vi "Drive_Execute.vi"() -> ()   [LabVIEW 2018]
uses:
  Drive_Control_Type.ctl
  <vilib>/Rock Robotics/WPI/ThirdParty/Phoenix-LabVIEW/Motor Controller/Controls/CTRE_Phoenix_MotorControl_ControlMode.ctl
  Global_Variables/Drive_Globals.vi
  Global_Variables/Sensor_Values.vi
  Global_Variables/Climb_Globals.vi
  Global_Variables/Kinematic_Globals.vi
  <vilib>/Utility/file.llb/Write Delimited Spreadsheet (DBL).vi
panel:
  in  "kP_Turn_Target":dbl
  in  "Kd":dbl
  in  "Ki":dbl
  in  "Kp":dbl=0.012
  in  "Turn_Adjust":dbl=0.015
  in  "Max_Linear_Speed":dbl=18.0
  in  "Max_Rotational_Speed":dbl=4.15
  out "Wheel_Speeds":cluster{dbl, dbl, dbl, dbl}(graph)
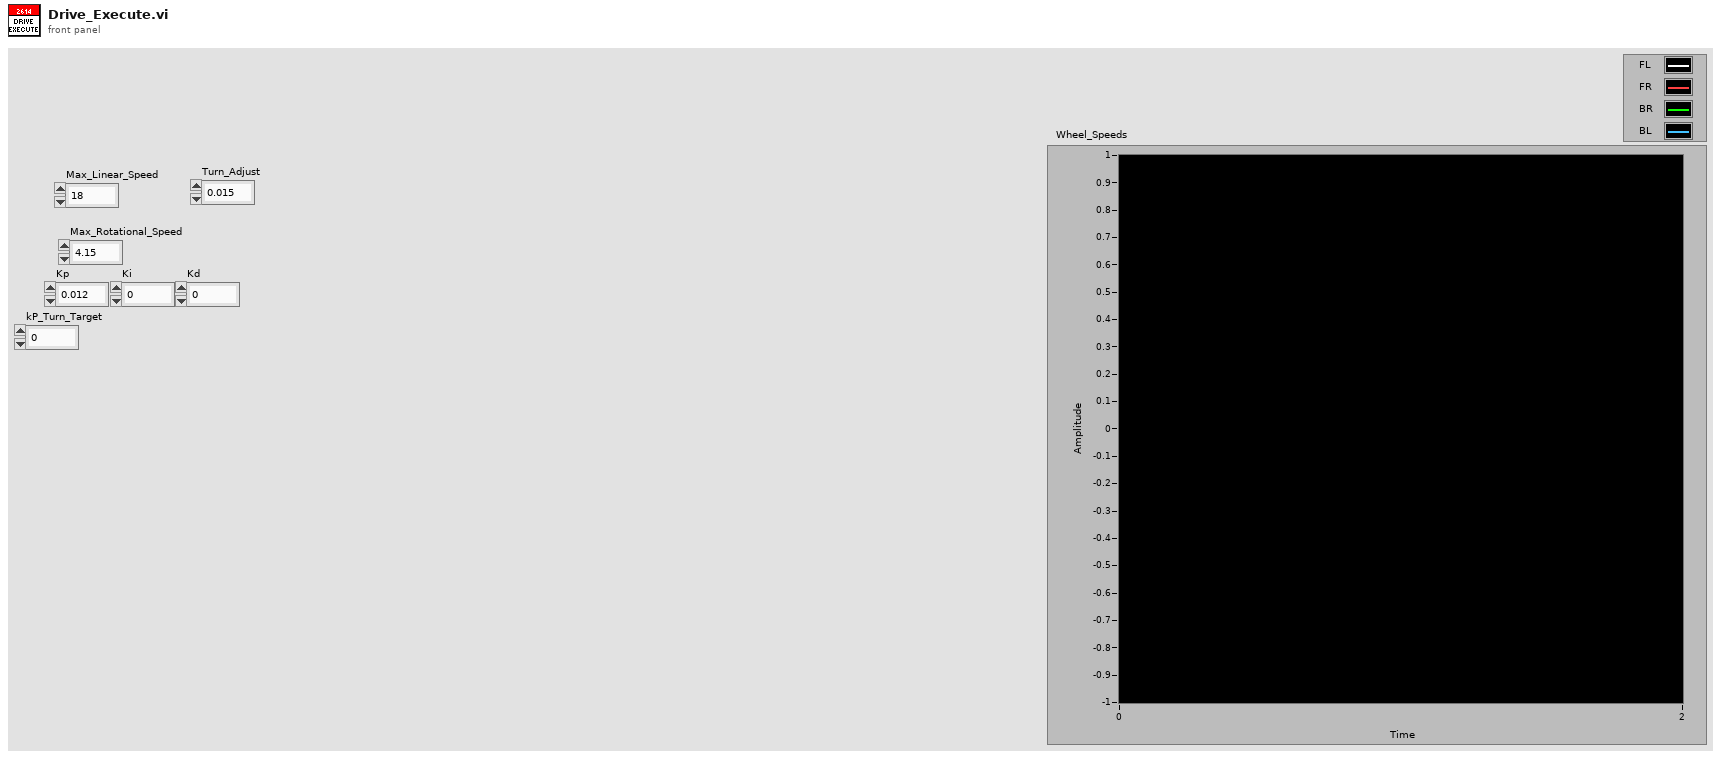
[diagram p1: front panel]
types:
  T1 = typedef "WPI_MotorControlDeviceRef.ctl" = cluster{"DeviceStatus":errorcluster, "Type":T2, "PWM":cluster{"PWM Channel":T3, "DeadBand":T4}, "CAN":cluster{"Device Number":u8, "SetOutput VI Ref":variant, "GetOutput VI Ref":variant, "Enable VI Ref":variant, "Disable VI Ref":variant, "Data":variant}, "Invert":bool, "DIO PWM":cluster{"PWM \"Enable\" Channel":T3, "DIOChannel":T5, "PWM Rate":dbl}}
  T2 = typedef "WPI_MotorControlType.ctl" = enum16{"PWM", "CAN", "DIO PWM"}
  T3 = typedef "FPGA_DIOPWMChannel.ctl" = enum8{"PWM 0", "PWM 1", "PWM 2", "PWM 3", "PWM 4", "PWM 5", "PWM 6", "PWM 7", "PWM 8", "PWM 9", "PWM MXP 0", "PWM MXP 1", "PWM MXP 2", "PWM MXP 3", "PWM MXP 4", "PWM MXP 5", "PWM MXP 6", "PWM MXP 7", "PWM MXP 8", "PWM MXP 9", "Invalid"}
  T4 = typedef "WPI_PWMDeadband.ctl" = cluster{"Name":string, "maxPositivePwm":i32, "minPositivePwm":i32, "centerPwm":i32, "maxNegativePwm":i32, "minNegativePwm":i32, "angularRange":u16}
  T5 = typedef "FPGA_DIOChannel.ctl" = enum8{"DIO 0", "DIO 1", "DIO 2", "DIO 3", "DIO 4", "DIO 5", "DIO 6", "DIO 7", "DIO 8", "DIO 9", "DIO MXP 0", "DIO MXP 1", "DIO MXP 2", "DIO MXP 3", "DIO MXP 4", "DIO MXP 5", "DIO MXP 6", "DIO MXP 7", "DIO MXP 8", "DIO MXP 9", "DIO MXP 10", "DIO MXP 11", "DIO MXP 12", "DIO MXP 13", "DIO MXP 14", "DIO MXP 15", "SPI Port CS1", "SPI Port CS2", "SPI Port CS3", "SPI Port MISO", "SPI Port MOSI", "Invalid"}
  T6 = typedef "CTRE_PigeonIMU_DeviceRef.ctl" = cluster{"DeviceStatus":errorcluster, "Device Number":u8, "Type":T7, "Device ID":u32, "Handle":u64, "UsageFrame":u32, "Library Path":path}
  T7 = typedef "CTRE_PigeonIMU_ConnectionType.ctl" = u32
  T8 = typedef "Drive_Control_Type.ctl" = enum16{"No_Op", "Write_FL_Position", "Write_FR_Position", "Write_BL_Position", "Write_BR_Position", "Set_Encoder_Positions", "Fieldcentric_PercentVBus", "Fieldcentric", "Robotcentric", "Reset_Gyro", "FR_Wheel", "FL_Wheel", "BR_Wheel", "BL_Wheel", "Drive_Onto_Platform", "Manual_Wheel_Control", "Distance", "Turn_To_Heading", "Turn_To_Target", "Drive_To_Target", "Zero", "Auto_Target", "Drive_Over_Platform", "Heading_Lock", "Time"}
  T9 = typedef "Drive_Notifier.ctl" = cluster{"Drive Control List":T8, "Front/Back":dbl, "Left/Right":dbl, "Turn":dbl, "Test_Joy_Y":dbl, "Test_Joy_X":dbl, "Set Wheel Encoder Positions":bool, "Robotcentric":bool, "Reset Gyro":bool, "Rotate Front Right":bool, "Rotate Front Left":bool, "Rotate Back Right":bool, "Rotate Back Left":bool, "Write_Encoder_Positions":bool, "Climb_Advance":bool, "Parameter_One":dbl, "Parameter_Two":dbl, "Parameter_Three":dbl, "Parameter_Four":dbl, "Drive_Notifier":refnum<notifier>, "Step":i32, "Climb_Reverse":bool, "Auto_Target":bool}
  T10 = typedef "CTRE_Phoenix_MotorControl_ControlMode.ctl" = u16
  T11 = cluster{"FL_Out":dbl, "FR_Out":dbl, "BL_Out":dbl, "BR_Out":dbl}
  T12 = cluster{"offsetAngle H":dbl, "offsetAngle V":dbl, "area":dbl, "skew":dbl}
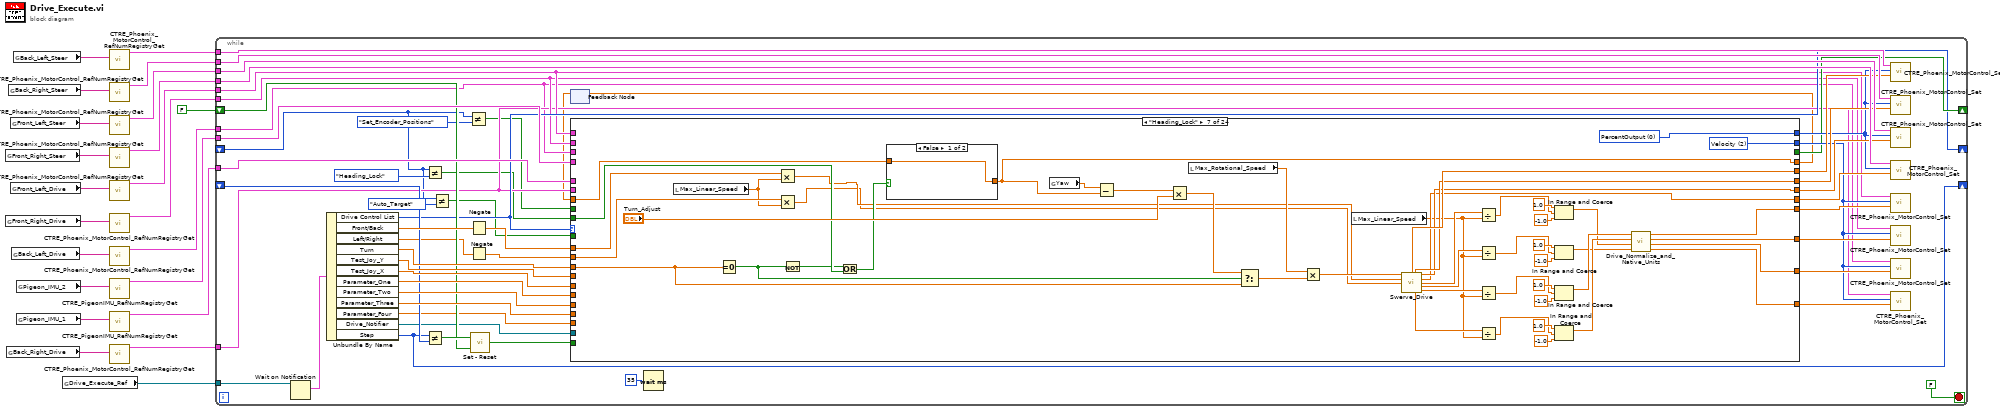
[diagram p0: block diagram]
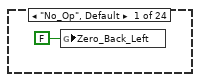
[diagram p2: hidden frame]
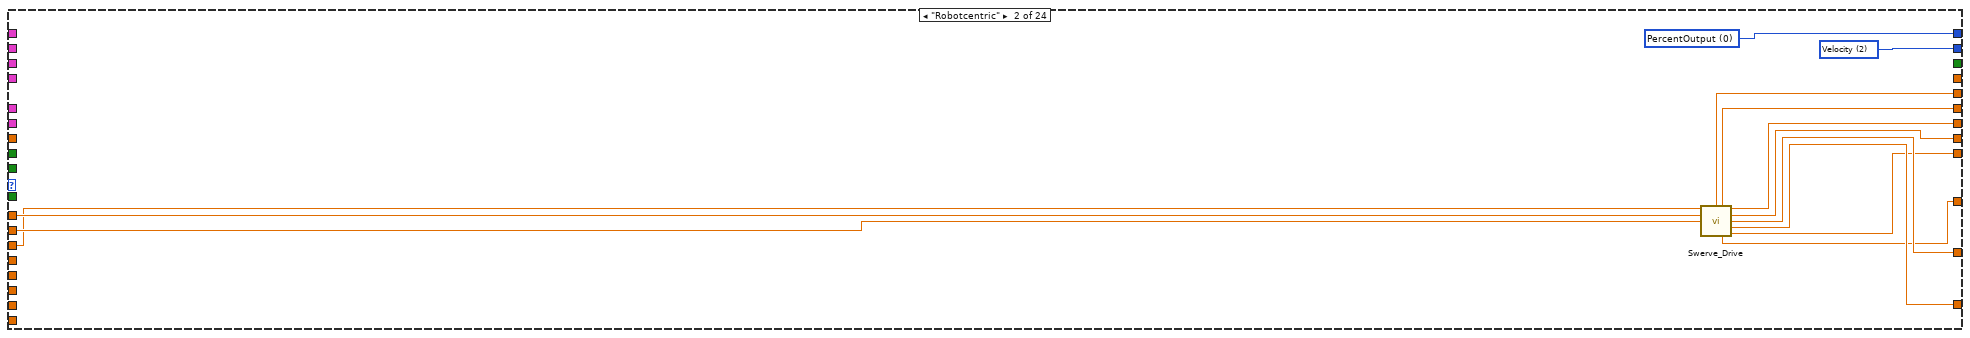
[diagram p3: hidden frame]
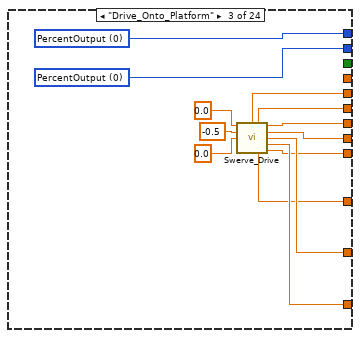
[diagram p4: hidden frame]
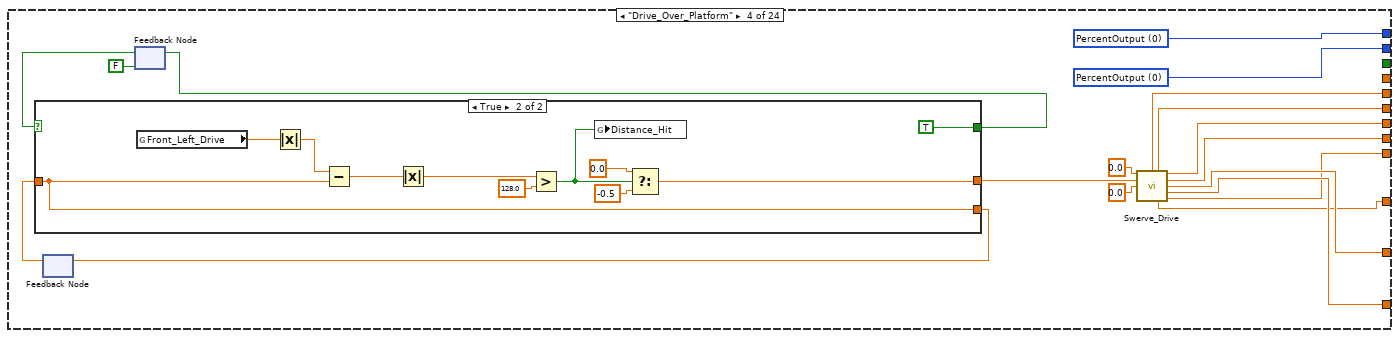
[diagram p5: hidden frame]
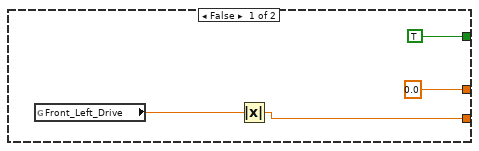
[diagram p6: hidden frame]
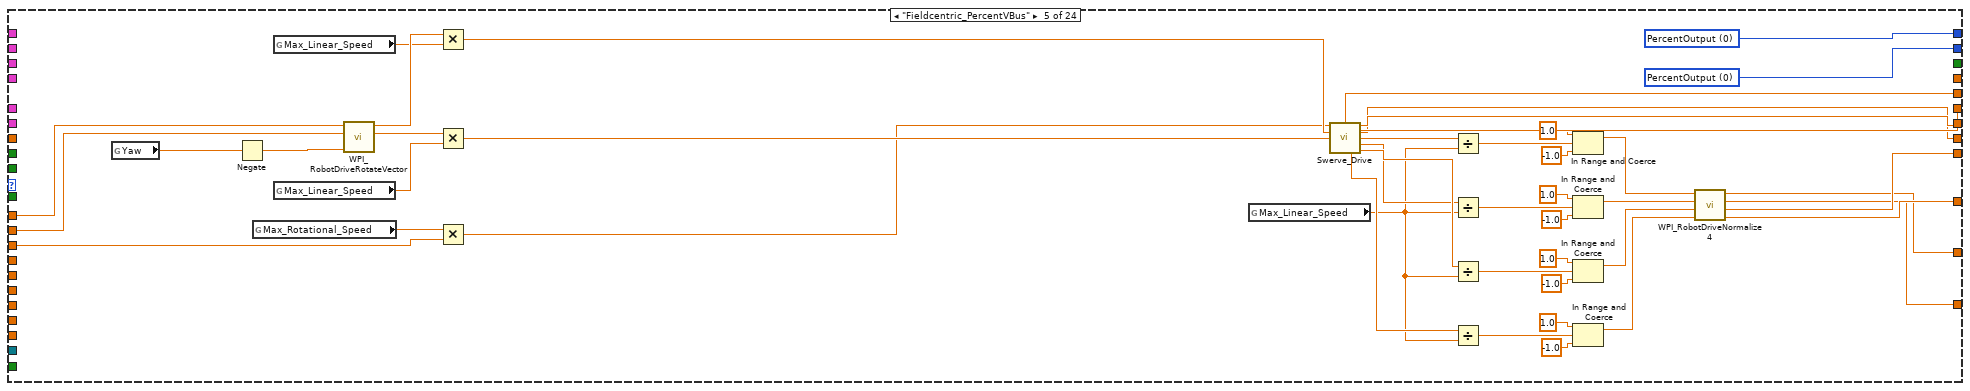
[diagram p7: hidden frame]
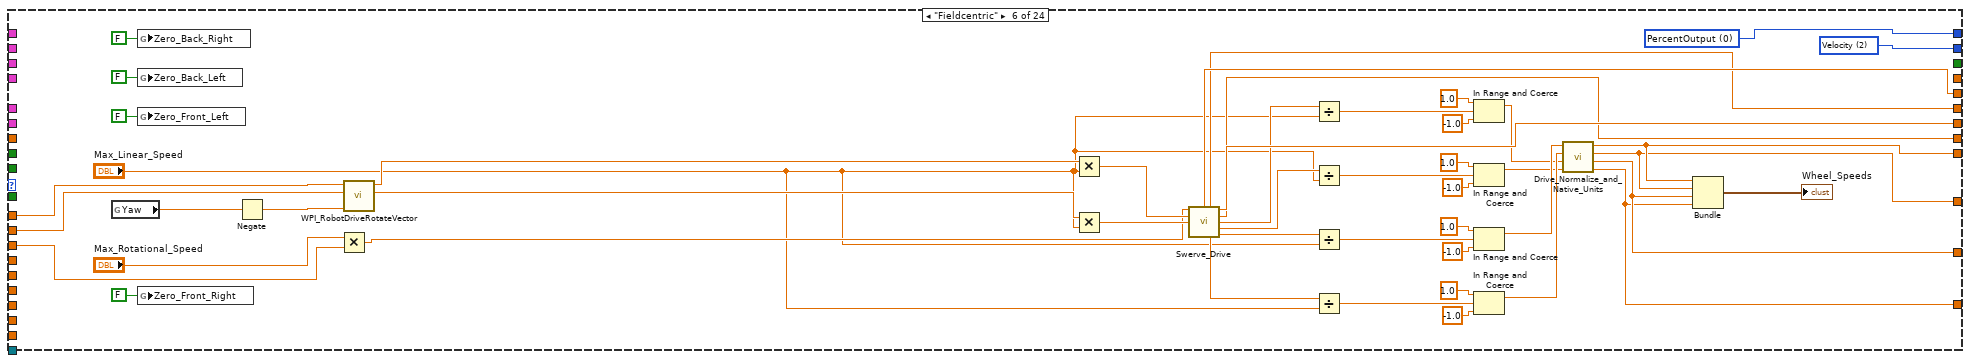
[diagram p8: hidden frame]
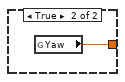
[diagram p9: hidden frame]
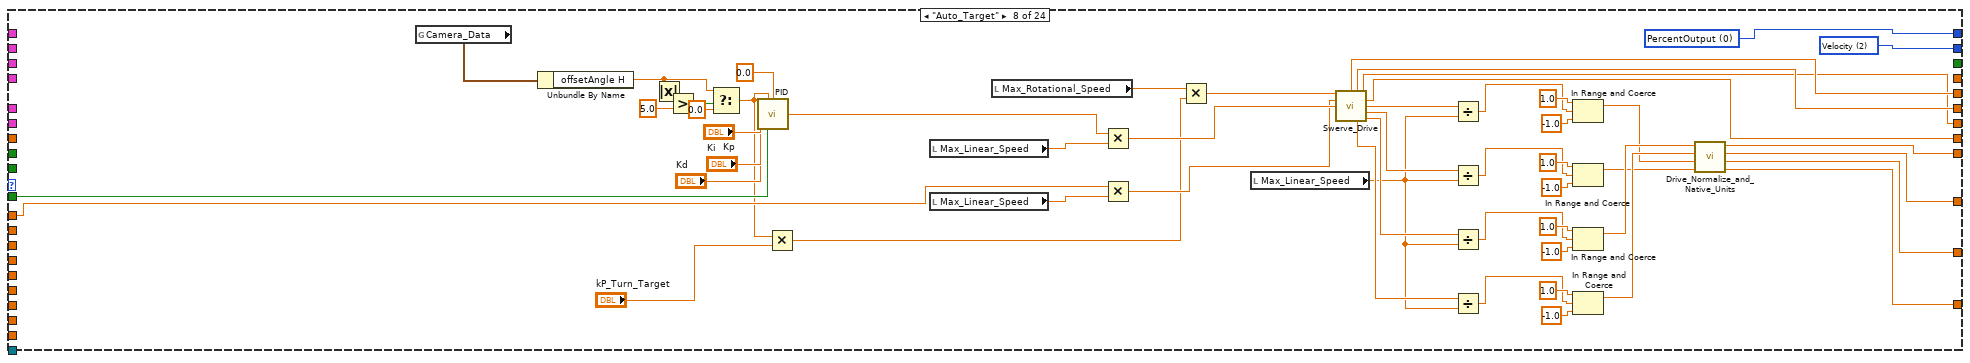
[diagram p10: hidden frame]
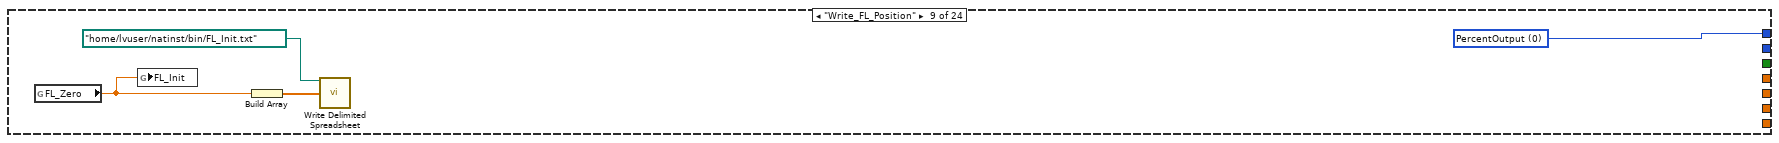
[diagram p11: hidden frame]
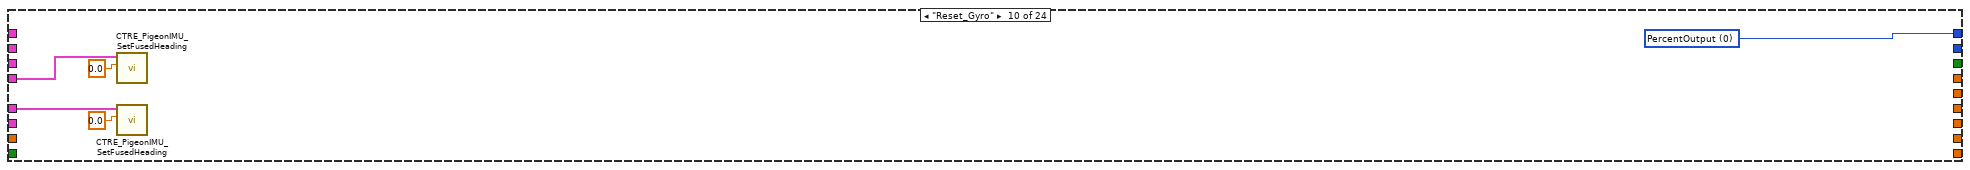
[diagram p12: hidden frame]
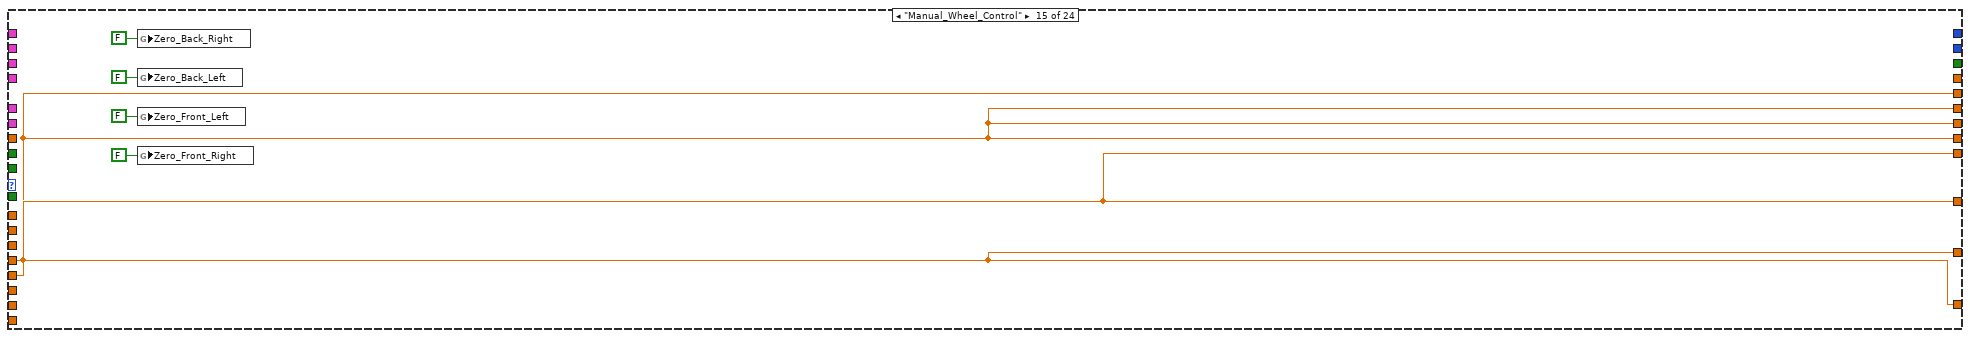
[diagram p17: hidden frame]
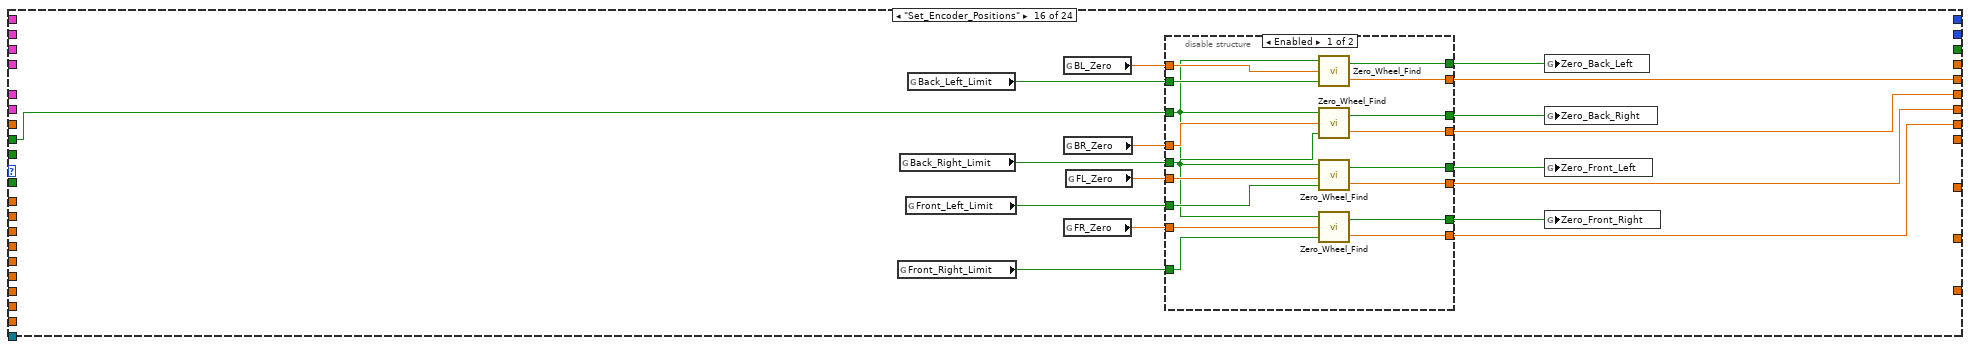
[diagram p18: hidden frame]
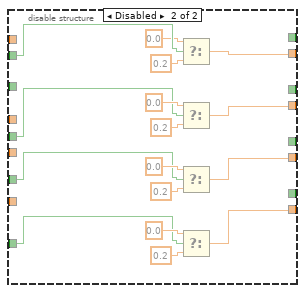
[diagram p19: hidden frame]
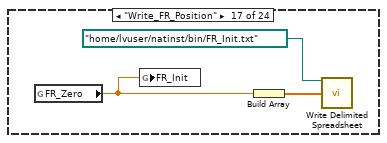
[diagram p20: hidden frame]
diagram:
  n1 = global read "Drive_Globals.vi" "Front_Right_Steer"() -> (w7:string)
  n2 = global read "Drive_Globals.vi" "Front_Right_Drive"() -> (w12:string)
  n3 = global read "Drive_Globals.vi" "Back_Right_Drive"() -> (w10:string)
  n4 = global read "Drive_Globals.vi" "Back_Right_Steer"() -> (w5:string)
  n5 = global read "Drive_Globals.vi" "Front_Left_Steer"() -> (w6:string)
  n6 = global read "Drive_Globals.vi" "Front_Left_Drive"() -> (w11:string)
  n7 = global read "Drive_Globals.vi" "Back_Left_Drive"() -> (w9:string)
  n8 = global read "Drive_Globals.vi" "Back_Left_Steer"() -> (w8:string)
  n9 = global read "Drive_Globals.vi" "Pigeon_IMU_2"() -> (w3:string)
  n10 = global read "Drive_Globals.vi" "Pigeon_IMU_1"() -> (w4:string)
  n11 = global read "Drive_Globals.vi" "Drive_Execute_Ref"() -> (w22:refnum<notifier>)
  n12 = call <vilib>:"CTRE_Phoenix_MotorControl_RefNumRegistryGet.vi"("refnum name"=w8) -> ("PhoenixMotorControlDevRef"=w17:T1)  [unwired: 9 in, 1 out]
  n13 = call <vilib>:"CTRE_Phoenix_MotorControl_RefNumRegistryGet.vi"("refnum name"=w5) -> ("PhoenixMotorControlDevRef"=w14:T1)  [unwired: 9 in, 1 out]
  n14 = call <vilib>:"CTRE_Phoenix_MotorControl_RefNumRegistryGet.vi"("refnum name"=w6) -> ("PhoenixMotorControlDevRef"=w15:T1)  [unwired: 9 in, 1 out]
  n15 = call <vilib>:"CTRE_Phoenix_MotorControl_RefNumRegistryGet.vi"("refnum name"=w7) -> ("PhoenixMotorControlDevRef"=w16:T1)  [unwired: 9 in, 1 out]
  n16 = call <vilib>:"CTRE_Phoenix_MotorControl_RefNumRegistryGet.vi"("refnum name"=w11) -> ("PhoenixMotorControlDevRef"=w20:T1)  [unwired: 9 in, 1 out]
  n17 = call <vilib>:"CTRE_Phoenix_MotorControl_RefNumRegistryGet.vi"("refnum name"=w12) -> ("PhoenixMotorControlDevRef"=w21:T1)  [unwired: 9 in, 1 out]
  n18 = call <vilib>:"CTRE_Phoenix_MotorControl_RefNumRegistryGet.vi"("refnum name"=w9) -> ("PhoenixMotorControlDevRef"=w19:T1)  [unwired: 9 in, 1 out]
  n19 = call <vilib>:"CTRE_PigeonIMU_RefNumRegistryGet.vi"("refnum name"=w3) -> ("PigeonIMUDevRef"=w2:T6)  [unwired: 9 in, 1 out]
  n20 = call <vilib>:"CTRE_PigeonIMU_RefNumRegistryGet.vi"("refnum name"=w4) -> ("PigeonIMUDevRef"=w13:T6)  [unwired: 9 in, 1 out]
  n21 = call <vilib>:"CTRE_Phoenix_MotorControl_RefNumRegistryGet.vi"("refnum name"=w10) -> ("PhoenixMotorControlDevRef"=w18:T1)  [unwired: 9 in, 1 out]
  n22 = while {
    tunnel: w22 -> [w54]
    tunnel: w21 -> [w36]
    tunnel: w20 -> [w37]
    tunnel: w19 -> [w34]
    tunnel: w18 -> [w35]
    tunnel: w14 -> [w71]
    tunnel: w17 -> [w58]
    tunnel: w16 -> [w70]
    tunnel: w15 -> [w69]
    tunnel: w13 -> [w57]
    tunnel: w2 -> [w51]
    shift-right: [w38] -> _
    shift-left: _ -> [w25]
    shift-right: [w43] -> _
    shift-left: _ -> [w44]
    shift-right: [w47] -> _
    shift-left: FALSE ("Reinit") -> [w45]
    stop <- FALSE stop-if-true
    n23 = Wait on Notification(notifier=w54) -> (notification=w40:T9)  [unwired: 3 in, 3 out]
    n24 = Unbundle By Name(w40) -> ("Drive Control List"=w38:T8, "Front/Back"=w72:dbl, "Left/Right"=w33:dbl, "Turn"=w68:dbl, "Test_Joy_Y"=w56:dbl, "Test_Joy_X"=w53:dbl, "Parameter_One"=w50:dbl, "Parameter_Two"=w48:dbl, "Parameter_Three"=w49:dbl, "Parameter_Four"=w39:dbl, "Drive_Notifier"=w41:refnum<notifier>, "Step"=w43:i32)
    n25 = Not Equal?(x=w25, y=Drive_Control_Type."Heading_Lock") -> (x != y?=w26:bool)
    n26 = Not Equal?(x=w43, y=w44) -> (x != y?=w46:bool)
    n27 = Not Equal?(x=w25, y=Drive_Control_Type."Auto_Target") -> (x != y?=w23:bool)
    n28 = Not Equal?(x=w25, y=Drive_Control_Type."Set_Encoder_Positions") -> (x != y?=w30:bool)
    n29 = Negate(x=w72) -> (-x=w52:dbl)
    n30 = Negate(x=w33) -> (-x=w32:dbl)
    n31 = call "Set - Reset.vi"("Reset"=w45, "Set"=w46) -> ("Output"=w42:bool)
    n32 = feedback #1() -> (w29:dbl)  [unwired: 1 in]
    n33 = case shown="\"Heading_Lock\"" w38 {
      tunnel: w52 -> [_ w78 _ _ w171 w218 w243 w285 _ _ _ _ _ _ _ _ _ _ _ _ _ _ _ _]
      tunnel: w32 -> [_ w79 _ _ w170 w217 w242 _ _ _ _ _ _ _ _ _ _ _ _ _ _ _ _ _]
      tunnel: w68 -> [_ w76 _ _ w143 w194 w234 _ _ _ _ _ _ _ _ _ _ _ _ _ _ _ _ _]
      tunnel: [_ w87 w100 w118 w177 w224 w274 w329 _ _ _ _ _ w346 w352 w370 _ _ _ w427 w452 w464 w478 w495] -> w67
      tunnel: [_ w83 w96 w114 w135 w186 w246 w301 _ _ _ _ _ w347 w353 _ _ _ _ w418 w445 w460 w474 w491] -> w66
      tunnel: [_ w86 w99 w117 w176 w223 w273 w328 _ _ _ _ w345 _ w352 w363 _ _ _ w426 w451 w463 w477 w494] -> w65
      tunnel: [_ w82 w95 w113 w136 w185 w245 w300 _ _ _ _ w344 _ w353 _ _ _ _ w420 w447 w459 w473 w490] -> w64
      tunnel: [_ w84 w97 w115 w174 w221 w271 w326 _ _ w341 _ _ _ w352 w354 _ _ _ w424 w449 w461 w475 w492] -> w63
      tunnel: [_ w80 w93 w111 w138 w187 w247 w302 _ _ w340 _ _ _ w353 _ _ _ _ w414 w441 w457 w471 w488] -> w62
      tunnel: [_ w85 w98 w116 w175 w222 w272 w327 _ _ _ w342 _ _ w352 w359 _ _ _ w425 w450 w462 w476 w493] -> w61
      tunnel: [_ w81 w94 w112 w137 w188 w248 w303 _ _ _ w343 _ _ w353 _ _ _ _ w416 w443 w458 w472 w489] -> w60
      tunnel: [_ w88 w101 w119 w178 w225 w275 w330 w334 w339 _ _ _ _ _ _ _ _ _ _ _ _ _ _] -> w59
      tunnel: w57 -> [_ _ _ _ _ _ _ _ _ w338 _ _ _ _ _ _ _ _ _ _ _ _ _ _]
      tunnel: w56 -> [_ _ _ _ _ _ _ _ _ _ w340 w343 w344 w347 w353 _ _ _ _ _ _ _ _ _]
      tunnel: [_ w77 w92 w110 w173 w220 w270 w325 _ _ _ _ _ _ _ _ _ _ _ w413 w440 w454 _ w486] -> w55
      tunnel: w53 -> [_ _ _ _ _ _ _ _ _ _ w341 w342 w345 w346 w352 _ _ _ _ _ _ _ _ _]
      tunnel: w51 -> [_ _ _ _ _ _ _ _ _ w335 _ _ _ _ _ _ _ _ _ _ _ _ _ _]
      tunnel: w50 -> [_ _ _ _ _ _ _ _ _ _ _ _ _ _ _ _ _ _ _ _ w433 w455 _ w485]
      tunnel: w49 -> [_ _ _ _ _ _ _ _ _ _ _ _ _ _ _ _ _ _ _ w422 _ _ _ _]
      tunnel: w48 -> [_ _ _ _ _ _ _ _ _ _ _ _ _ _ _ _ _ _ _ _ w434 _ _ w484]
      tunnel: [_ _ _ _ _ _ _ _ _ _ _ _ _ _ _ _ _ _ _ w432 w437 w469 w483 w500] -> w47
      tunnel: w42 -> [_ _ _ _ _ _ _ _ _ _ _ _ _ _ _ _ _ _ _ w431 w436 w468 w482 w499]
      tunnel: w41 -> [_ _ _ _ _ _ _ _ _ _ _ _ _ _ _ _ _ _ _ w429 w453 w466 w480 w497]
      tunnel: w39 -> [_ _ _ _ _ _ _ _ _ _ _ _ _ _ _ _ _ _ _ w423 w435 w456 w470 w487]
      tunnel: w37 -> [_ _ _ _ _ _ _ _ _ _ _ _ _ _ _ _ _ _ _ _ _ _ _ _]
      tunnel: w36 -> [_ _ _ _ _ _ _ _ _ _ _ _ _ _ _ _ _ _ _ _ _ _ _ _]
      tunnel: w35 -> [_ _ _ _ _ _ _ _ _ _ _ _ _ _ _ _ _ _ _ _ _ _ _ _]
      tunnel: w34 -> [_ _ _ _ _ _ _ _ _ _ _ _ _ _ _ _ _ _ _ _ _ _ _ _]
      tunnel: w30 -> [_ _ _ _ _ _ _ _ _ _ _ _ _ _ _ w355 _ _ _ _ _ _ _ _]
      tunnel: w29 -> [_ _ _ _ _ _ w236 _ _ _ _ _ _ _ _ _ _ _ _ _ _ _ _ _]
      tunnel: w26 -> [_ _ _ _ _ _ w237 _ _ _ _ _ _ _ _ _ _ _ _ _ _ _ _ _]
      tunnel: [_ _ _ _ _ _ w235 _ _ _ _ _ _ _ _ _ _ _ _ _ _ _ _ _] -> w27
      tunnel: w23 -> [_ _ _ _ _ _ _ w297 _ _ _ _ _ _ _ _ _ _ _ _ _ _ _ _]
      frame "No_Op", Default {
        n34 = global write "Drive_Globals.vi" "Zero_Back_Left"(FALSE ("Zero_Back_Left")) -> ()
      }
      frame "Robotcentric" {
        w77 = T10 2 items=["PercentOutput"=0, "Position"=1, "Velocity"=2, "Current"=3, "Follower"=5, "MotionProfile"=6, "MotionMagic"=7, "MotionMagicArc"=8, "MotionProfileArc"=10, "Disabled"=15] ("Control Mode")
        w88 = T10 0 items=["PercentOutput"=0, "Position"=1, "Velocity"=2, "Current"=3, "Follower"=5, "MotionProfile"=6, "MotionMagic"=7, "MotionMagicArc"=8, "MotionProfileArc"=10, "Disabled"=15] ("Control Mode")
        n35 = call "Swerve_Drive.vi"("Z"=w76, "Y"=w78, "X"=w79) -> ("Back Left Spin Speed"=w87:dbl, "Back Right Spin Speed"=w86:dbl, "Front Left Spin Speed"=w85:dbl, "Front Right Spin Speed"=w84:dbl, "Back Left Motor Power"=w83:dbl, "Back Right Motor Power"=w82:dbl, "Front Right Motor Power"=w80:dbl, "Front Left Motor Power"=w81:dbl)  [unwired: 5 in]
      }
      frame "Drive_Onto_Platform" {
        w92 = T10 0 items=["PercentOutput"=0, "Position"=1, "Velocity"=2, "Current"=3, "Follower"=5, "MotionProfile"=6, "MotionMagic"=7, "MotionMagicArc"=8, "MotionProfileArc"=10, "Disabled"=15] ("Control Mode")
        w101 = T10 0 items=["PercentOutput"=0, "Position"=1, "Velocity"=2, "Current"=3, "Follower"=5, "MotionProfile"=6, "MotionMagic"=7, "MotionMagicArc"=8, "MotionProfileArc"=10, "Disabled"=15] ("Control Mode")
        n36 = call "Swerve_Drive.vi"("Z"=0.0, "Y"=-0.5, "X"=0.0) -> ("Back Left Spin Speed"=w100:dbl, "Back Right Spin Speed"=w99:dbl, "Front Left Spin Speed"=w98:dbl, "Front Right Spin Speed"=w97:dbl, "Back Left Motor Power"=w96:dbl, "Back Right Motor Power"=w95:dbl, "Front Right Motor Power"=w93:dbl, "Front Left Motor Power"=w94:dbl)  [unwired: 5 in]
      }
      frame "Drive_Over_Platform" {
        w110 = T10 0 items=["PercentOutput"=0, "Position"=1, "Velocity"=2, "Current"=3, "Follower"=5, "MotionProfile"=6, "MotionMagic"=7, "MotionMagicArc"=8, "MotionProfileArc"=10, "Disabled"=15] ("Control Mode")
        w119 = T10 0 items=["PercentOutput"=0, "Position"=1, "Velocity"=2, "Current"=3, "Follower"=5, "MotionProfile"=6, "MotionMagic"=7, "MotionMagicArc"=8, "MotionProfileArc"=10, "Disabled"=15] ("Control Mode")
        n37 = feedback #2() -> (w102:dbl)  [unwired: 1 in]
        n38 = feedback #3(FALSE) -> (w107:bool)
        n39 = case shown="True" w107 {
          tunnel: [TRUE TRUE] -> w105
          tunnel: [0.0 ("Y") w126] -> w104
          tunnel: [w120 w128] -> w103
          tunnel: w102 -> [_ w128]
          frame False {
            n40 = global read "Sensor_Values.vi" "Front_Left_Drive"() -> (w121:dbl)
            n41 = Absolute Value(x=w121) -> (abs(x)=w120:dbl)
          }
          frame True {
            n42 = global read "Sensor_Values.vi" "Front_Left_Drive"() -> (w133:dbl)
            n43 = Absolute Value(x=w133) -> (abs(x)=w132:dbl)
            n44 = Subtract(x=w132, y=w128) -> (x-y=w131:dbl)
            n45 = Absolute Value(x=w131) -> (abs(x)=w130:dbl)
            n46 = Greater?(x=w130, y=128.0) -> (0:w124:bool)
            n47 = global write "Climb_Globals.vi" "Distance_Hit"(w124) -> ()
            n48 = Select(t=0.0, s=w124, f=-0.5 ("Y")) -> (s? t:f=w126:dbl)
          }
        }
        n49 = feedback-in #2(w103) -> ()
        n50 = feedback-in #3(w105) -> ()
        n51 = call "Swerve_Drive.vi"("Z"=0.0, "Y"=w104, "X"=0.0) -> ("Back Left Spin Speed"=w118:dbl, "Back Right Spin Speed"=w117:dbl, "Front Left Spin Speed"=w116:dbl, "Front Right Spin Speed"=w115:dbl, "Back Left Motor Power"=w114:dbl, "Back Right Motor Power"=w113:dbl, "Front Right Motor Power"=w111:dbl, "Front Left Motor Power"=w112:dbl)  [unwired: 5 in]
      }
      frame "Fieldcentric_PercentVBus" {
        w173 = T10 0 items=["PercentOutput"=0, "Position"=1, "Velocity"=2, "Current"=3, "Follower"=5, "MotionProfile"=6, "MotionMagic"=7, "MotionMagicArc"=8, "MotionProfileArc"=10, "Disabled"=15] ("Control Mode")
        w178 = T10 0 items=["PercentOutput"=0, "Position"=1, "Velocity"=2, "Current"=3, "Follower"=5, "MotionProfile"=6, "MotionMagic"=7, "MotionMagicArc"=8, "MotionProfileArc"=10, "Disabled"=15] ("Control Mode")
        n52 = global read "Sensor_Values.vi" "Yaw"() -> (w172:dbl)
        n53 = Negate(x=w172) -> (-x=w169:dbl)
        n54 = global read "Kinematic_Globals.vi" "Max_Rotational_Speed"() -> (w145:dbl)
        n55 = global read "Kinematic_Globals.vi" "Max_Linear_Speed"() -> (w146:dbl)
        n56 = global read "Kinematic_Globals.vi" "Max_Linear_Speed"() -> (w151:dbl)
        n57 = call <vilib>:"WPI_RobotDriveRotateVector.vi"("Angle"=w169, "X"=w170, "Y"=w171) -> ("X'"=w150:dbl, "Y'"=w147:dbl)  [unwired: 7 out]
        n58 = Multiply(x=w147, y=w146) -> (x*y=w148:dbl)
        n59 = Multiply(x=w150, y=w151) -> (x*y=w149:dbl)
        n60 = Multiply(x=w145, y=w143) -> (x*y=w144:dbl)
        n61 = global read "Kinematic_Globals.vi" "Max_Linear_Speed"() -> (w152:dbl)
        n62 = call "Swerve_Drive.vi"("Z"=w144, "Y"=w148, "X"=w149) -> ("Back Left Spin Speed"=w177:dbl, "Back Right Spin Speed"=w176:dbl, "Front Left Spin Speed"=w175:dbl, "Front Right Spin Speed"=w174:dbl, "Back Left Motor Power"=w153:dbl, "Back Right Motor Power"=w158:dbl, "Front Right Motor Power"=w161:dbl, "Front Left Motor Power"=w166:dbl)  [unwired: 5 in]
        n63 = Divide(x=w153, y=w152) -> (x/y=w155:dbl)
        n64 = Divide(x=w158, y=w152) -> (x/y=w154:dbl)
        n65 = Divide(x=w166, y=w152) -> (x/y=w165:dbl)
        n66 = Divide(x=w161, y=w152) -> (x/y=w162:dbl)
        n67 = In Range and Coerce(upper limit=1.0, x=w155, lower limit=-1.0) -> (coerced(x)=w139:dbl)  [unwired: 1 out]
        n68 = In Range and Coerce(upper limit=1.0, x=w154, lower limit=-1.0) -> (coerced(x)=w140:dbl)  [unwired: 1 out]
        n69 = In Range and Coerce(upper limit=1.0, x=w165, lower limit=-1.0) -> (coerced(x)=w141:dbl)  [unwired: 1 out]
        n70 = In Range and Coerce(upper limit=1.0, x=w162, lower limit=-1.0) -> (coerced(x)=w142:dbl)  [unwired: 1 out]
        n71 = call <vilib>:"WPI_RobotDriveNormalize 4.vi"("D"=w142, "C"=w141, "B"=w140, "A"=w139) -> ("D'"=w138:dbl, "C'"=w137:dbl, "B'"=w136:dbl, "A'"=w135:dbl)
      }
      frame "Fieldcentric" {
        w220 = T10 2 items=["PercentOutput"=0, "Position"=1, "Velocity"=2, "Current"=3, "Follower"=5, "MotionProfile"=6, "MotionMagic"=7, "MotionMagicArc"=8, "MotionProfileArc"=10, "Disabled"=15] ("Control Mode")
        w225 = T10 0 items=["PercentOutput"=0, "Position"=1, "Velocity"=2, "Current"=3, "Follower"=5, "MotionProfile"=6, "MotionMagic"=7, "MotionMagicArc"=8, "MotionProfileArc"=10, "Disabled"=15] ("Control Mode")
        n72 = global read "Sensor_Values.vi" "Yaw"() -> (w219:dbl)
        n73 = global write "Drive_Globals.vi" "Zero_Back_Right"(FALSE ("Zero_Back_Left")) -> ()
        n74 = global write "Drive_Globals.vi" "Zero_Back_Left"(FALSE ("Zero_Back_Left")) -> ()
        n75 = global write "Drive_Globals.vi" "Zero_Front_Left"(FALSE ("Zero_Back_Left")) -> ()
        n76 = global write "Drive_Globals.vi" "Zero_Front_Right"(FALSE ("Zero_Back_Left")) -> ()
        n77 = Negate(x=w219) -> (-x=w216:dbl)
        n78 = Multiply(x="Max_Rotational_Speed", y=w194) -> (x*y=w195:dbl)
        n79 = call <vilib>:"WPI_RobotDriveRotateVector.vi"("Angle"=w216, "X"=w217, "Y"=w218) -> ("X'"=w199:dbl, "Y'"=w196:dbl)  [unwired: 7 out]
        n80 = Multiply(x=w196, y="Max_Linear_Speed") -> (x*y=w197:dbl)
        n81 = Multiply(x=w199, y="Max_Linear_Speed") -> (x*y=w198:dbl)
        n82 = call "Swerve_Drive.vi"("Z"=w195, "Y"=w197, "X"=w198) -> ("Back Left Spin Speed"=w224:dbl, "Back Right Spin Speed"=w223:dbl, "Front Left Spin Speed"=w222:dbl, "Front Right Spin Speed"=w221:dbl, "Back Left Motor Power"=w200:dbl, "Back Right Motor Power"=w205:dbl, "Front Right Motor Power"=w208:dbl, "Front Left Motor Power"=w213:dbl)  [unwired: 5 in]
        n83 = Divide(x=w200, y="Max_Linear_Speed") -> (x/y=w202:dbl)
        n84 = Divide(x=w205, y="Max_Linear_Speed") -> (x/y=w201:dbl)
        n85 = Divide(x=w213, y="Max_Linear_Speed") -> (x/y=w212:dbl)
        n86 = Divide(x=w208, y="Max_Linear_Speed") -> (x/y=w209:dbl)
        n87 = In Range and Coerce(upper limit=1.0, x=w202, lower limit=-1.0) -> (coerced(x)=w190:dbl)  [unwired: 1 out]
        n88 = In Range and Coerce(upper limit=1.0, x=w201, lower limit=-1.0) -> (coerced(x)=w191:dbl)  [unwired: 1 out]
        n89 = In Range and Coerce(upper limit=1.0, x=w212, lower limit=-1.0) -> (coerced(x)=w193:dbl)  [unwired: 1 out]
        n90 = In Range and Coerce(upper limit=1.0, x=w209, lower limit=-1.0) -> (coerced(x)=w192:dbl)  [unwired: 1 out]
        n91 = call "Drive_Normalize_and_Native_Units.vi"("BR"=w191, "BL"=w190, "FR"=w192, "FL"=w193) -> ("BR_Out"=w185:dbl, "BL_Out"=w186:dbl, "FR_Out"=w187:dbl, "FL_Out"=w188:dbl)
        n92 = Bundle("FL_Out"=w188, "FR_Out"=w187, "BL_Out"=w186, "BR_Out"=w185) -> (→"Wheel_Speeds":T11)  [unwired: 1 in]
      }
      frame "Heading_Lock" {
        w270 = T10 2 items=["PercentOutput"=0, "Position"=1, "Velocity"=2, "Current"=3, "Follower"=5, "MotionProfile"=6, "MotionMagic"=7, "MotionMagicArc"=8, "MotionProfileArc"=10, "Disabled"=15] ("Control Mode")
        w275 = T10 0 items=["PercentOutput"=0, "Position"=1, "Velocity"=2, "Current"=3, "Follower"=5, "MotionProfile"=6, "MotionMagic"=7, "MotionMagicArc"=8, "MotionProfileArc"=10, "Disabled"=15] ("Control Mode")
        n93 = local read "Max_Linear_Speed"() -> (w228:dbl)
        n94 = Equal To 0?(x=w234) -> (x = 0?=w231:bool)
        n95 = Multiply(x=w243, y=w228) -> (x*y=w227:dbl)
        n96 = Multiply(x=w242, y=w228) -> (x*y=w226:dbl)
        n97 = Not(x=w231) -> (.not. x?=w230:bool)
        n98 = Or(x=w230, y=w237) -> (x .or. y?=w232:bool)
        n99 = case shown="False" w232 {
          tunnel: [w276 w277] -> w235
          tunnel: w236 -> [w276 _]
          frame False {
          }
          frame True {
            n100 = global read "Sensor_Values.vi" "Yaw"() -> (w277:dbl)
          }
        }
        n101 = global read "Sensor_Values.vi" "Yaw"() -> (w240:dbl)
        n102 = Subtract(x=w240, y=w235) -> (x-y=w239:dbl)
        n103 = Multiply(x=w239, y="Turn_Adjust") -> (x*y=w241:dbl)
        n104 = local read "Max_Rotational_Speed"() -> (w244:dbl)
        n105 = Select(t=w241, s=w231, f=w234) -> (s? t:f=w233:dbl)
        n106 = Multiply(x=w244, y=w233) -> (x*y=w253:dbl)
        n107 = local read "Max_Linear_Speed"() -> (w229:dbl)
        n108 = call "Swerve_Drive.vi"("Z"=w253, "Y"=w227, "X"=w226) -> ("Back Left Spin Speed"=w274:dbl, "Back Right Spin Speed"=w273:dbl, "Front Left Spin Speed"=w272:dbl, "Front Right Spin Speed"=w271:dbl, "Back Left Motor Power"=w254:dbl, "Back Right Motor Power"=w259:dbl, "Front Right Motor Power"=w262:dbl, "Front Left Motor Power"=w267:dbl)  [unwired: 5 in]
        n109 = Divide(x=w254, y=w229) -> (x/y=w256:dbl)
        n110 = Divide(x=w259, y=w229) -> (x/y=w255:dbl)
        n111 = Divide(x=w267, y=w229) -> (x/y=w266:dbl)
        n112 = Divide(x=w262, y=w229) -> (x/y=w263:dbl)
        n113 = In Range and Coerce(upper limit=1.0, x=w256, lower limit=-1.0) -> (coerced(x)=w249:dbl)  [unwired: 1 out]
        n114 = In Range and Coerce(upper limit=1.0, x=w255, lower limit=-1.0) -> (coerced(x)=w250:dbl)  [unwired: 1 out]
        n115 = In Range and Coerce(upper limit=1.0, x=w266, lower limit=-1.0) -> (coerced(x)=w252:dbl)  [unwired: 1 out]
        n116 = In Range and Coerce(upper limit=1.0, x=w263, lower limit=-1.0) -> (coerced(x)=w251:dbl)  [unwired: 1 out]
        n117 = call "Drive_Normalize_and_Native_Units.vi"("BR"=w250, "BL"=w249, "FR"=w251, "FL"=w252) -> ("BR_Out"=w245:dbl, "BL_Out"=w246:dbl, "FR_Out"=w247:dbl, "FL_Out"=w248:dbl)
      }
      frame "Auto_Target" {
        w325 = T10 2 items=["PercentOutput"=0, "Position"=1, "Velocity"=2, "Current"=3, "Follower"=5, "MotionProfile"=6, "MotionMagic"=7, "MotionMagicArc"=8, "MotionProfileArc"=10, "Disabled"=15] ("Control Mode")
        w330 = T10 0 items=["PercentOutput"=0, "Position"=1, "Velocity"=2, "Current"=3, "Follower"=5, "MotionProfile"=6, "MotionMagic"=7, "MotionMagicArc"=8, "MotionProfileArc"=10, "Disabled"=15] ("Control Mode")
        n118 = global read "Sensor_Values.vi" "Camera_Data"() -> (w296:T12)
        n119 = Unbundle By Name(w296) -> ("offsetAngle H"=w291:dbl)
        n120 = Absolute Value(x=w291) -> (abs(x)=w293:dbl)
        n121 = Greater?(x=w293, y=5.0) -> (0:w292:bool)
        n122 = Select(t=w291, s=w292, f=0.0) -> (s? t:f=w280:dbl)
        n123 = call "PID.vi"("Kp"="Kp", "Process Variable"=w280, "Goal"=0.0, "Ki"="Ki", "Kd"="Kd", "Reinit"=w297) -> ("Command"=w289:dbl)  [unwired: 7 in, 2 out]
        n124 = Multiply(x=w280, y="kP_Turn_Target") -> (x*y=w279:dbl)
        n125 = local read "Max_Linear_Speed"() -> (w287:dbl)
        n126 = local read "Max_Linear_Speed"() -> (w286:dbl)
        n127 = local read "Max_Rotational_Speed"() -> (w299:dbl)
        n128 = Multiply(x=w289, y=w287) -> (x*y=w288:dbl)
        n129 = Multiply(x=w285, y=w286) -> (x*y=w284:dbl)
        n130 = Multiply(x=w299, y=w279) -> (x*y=w308:dbl)
        n131 = local read "Max_Linear_Speed"() -> (w298:dbl)
        n132 = call "Swerve_Drive.vi"("Z"=w308, "Y"=w284, "X"=w288) -> ("Back Left Spin Speed"=w329:dbl, "Back Right Spin Speed"=w328:dbl, "Front Left Spin Speed"=w327:dbl, "Front Right Spin Speed"=w326:dbl, "Back Left Motor Power"=w309:dbl, "Back Right Motor Power"=w314:dbl, "Front Right Motor Power"=w317:dbl, "Front Left Motor Power"=w322:dbl)  [unwired: 5 in]
        n133 = Divide(x=w309, y=w298) -> (x/y=w311:dbl)
        n134 = Divide(x=w314, y=w298) -> (x/y=w310:dbl)
        n135 = Divide(x=w322, y=w298) -> (x/y=w321:dbl)
        n136 = Divide(x=w317, y=w298) -> (x/y=w318:dbl)
        n137 = In Range and Coerce(upper limit=1.0, x=w311, lower limit=-1.0) -> (coerced(x)=w304:dbl)  [unwired: 1 out]
        n138 = In Range and Coerce(upper limit=1.0, x=w310, lower limit=-1.0) -> (coerced(x)=w305:dbl)  [unwired: 1 out]
        n139 = In Range and Coerce(upper limit=1.0, x=w321, lower limit=-1.0) -> (coerced(x)=w307:dbl)  [unwired: 1 out]
        n140 = In Range and Coerce(upper limit=1.0, x=w318, lower limit=-1.0) -> (coerced(x)=w306:dbl)  [unwired: 1 out]
        n141 = call "Drive_Normalize_and_Native_Units.vi"("BR"=w305, "BL"=w304, "FR"=w306, "FL"=w307) -> ("BR_Out"=w300:dbl, "BL_Out"=w301:dbl, "FR_Out"=w302:dbl, "FL_Out"=w303:dbl)
      }
      frame "Write_FL_Position" {
        w334 = T10 0 items=["PercentOutput"=0, "Position"=1, "Velocity"=2, "Current"=3, "Follower"=5, "MotionProfile"=6, "MotionMagic"=7, "MotionMagicArc"=8, "MotionProfileArc"=10, "Disabled"=15] ("Control Mode")
        n142 = global read "Drive_Globals.vi" "FL_Zero"() -> (w331:dbl)
        n143 = global write "Drive_Globals.vi" "FL_Init"(w331) -> ()
        n144 = Build Array(w331) -> (w332:dbl[])
        n145 = call-poly <vilib>:"Write Delimited Spreadsheet.vi"("file path (dialog if empty)"=path "/home/lvuser/natinst/bin/FL_Init.txt" ("file (use dialog)"), "1D data"=w332) -> ()  [unwired: 12 in, 2 out]
      }
      frame "Reset_Gyro" {
        w339 = T10 0 items=["PercentOutput"=0, "Position"=1, "Velocity"=2, "Current"=3, "Follower"=5, "MotionProfile"=6, "MotionMagic"=7, "MotionMagicArc"=8, "MotionProfileArc"=10, "Disabled"=15] ("Control Mode")
        n146 = call <vilib>:"CTRE_PigeonIMU_SetFusedHeading.vi"("Value"=0.0, "PigeonIMUDevRef 2"=w335) -> ()  [unwired: 8 in, 2 out]
        n147 = call <vilib>:"CTRE_PigeonIMU_SetFusedHeading.vi"("Value"=0.0, "PigeonIMUDevRef 2"=w338) -> ()  [unwired: 8 in, 2 out]
      }
      frame "FR_Wheel" {
      }
      frame "FL_Wheel" {
      }
      frame "BR_Wheel" {
      }
      frame "BL_Wheel" {
      }
      frame "Manual_Wheel_Control" {
        n148 = global write "Drive_Globals.vi" "Zero_Back_Right"(FALSE ("Zero_Back_Left")) -> ()
        n149 = global write "Drive_Globals.vi" "Zero_Back_Left"(FALSE ("Zero_Back_Left")) -> ()
        n150 = global write "Drive_Globals.vi" "Zero_Front_Left"(FALSE ("Zero_Back_Left")) -> ()
        n151 = global write "Drive_Globals.vi" "Zero_Front_Right"(FALSE ("Zero_Back_Left")) -> ()
      }
      frame "Set_Encoder_Positions" {
        n152 = global read "Sensor_Values.vi" "Front_Right_Limit"() -> (w358:bool)
        n153 = global read "Sensor_Values.vi" "Back_Right_Limit"() -> (w366:bool)
        n154 = global read "Sensor_Values.vi" "Front_Left_Limit"() -> (w360:bool)
        n155 = global read "Sensor_Values.vi" "Back_Left_Limit"() -> (w367:bool)
        n156 = global read "Drive_Globals.vi" "BL_Zero"() -> (w368:dbl)
        n157 = global read "Drive_Globals.vi" "BR_Zero"() -> (w365:dbl)
        n158 = global read "Drive_Globals.vi" "FR_Zero"() -> (w356:dbl)
        n159 = global read "Drive_Globals.vi" "FL_Zero"() -> (w361:dbl)
        n160 = disable-structure shown="Enabled" {
          disable-tunnel: [w387 w400] -> w370
          disable-tunnel: [w386 _] -> w369
          disable-tunnel: w368 -> [w385 _]
          disable-tunnel: w367 -> [w384 w403]
          disable-tunnel: w366 -> [w383 w388]
          disable-tunnel: w365 -> [w382 _]
          disable-tunnel: [w381 _] -> w364
          disable-tunnel: [w380 w389] -> w363
          disable-tunnel: [w379 _] -> w362
          disable-tunnel: w361 -> [w378 _]
          disable-tunnel: w360 -> [w377 w391]
          disable-tunnel: [w376 w390] -> w359
          disable-tunnel: w358 -> [w375 w392]
          disable-tunnel: [w374 _] -> w357
          disable-tunnel: w356 -> [w373 _]
          disable-tunnel: w355 -> [w372 _]
          disable-tunnel: [w371 w393] -> w354
          frame Enabled {
            n161 = call "Zero_Wheel_Find.vi"("Limit"=w384, "Accum_Value"=w385, "Reinit"=w372) -> ("Wheel_Out"=w387:dbl, "Zeroed?"=w386:bool)
            n162 = call "Zero_Wheel_Find.vi"("Limit"=w383, "Accum_Value"=w382, "Reinit"=w372) -> ("Wheel_Out"=w380:dbl, "Zeroed?"=w381:bool)
            n163 = call "Zero_Wheel_Find.vi"("Limit"=w377, "Accum_Value"=w378, "Reinit"=w372) -> ("Wheel_Out"=w376:dbl, "Zeroed?"=w379:bool)
            n164 = call "Zero_Wheel_Find.vi"("Limit"=w375, "Accum_Value"=w373, "Reinit"=w372) -> ("Wheel_Out"=w371:dbl, "Zeroed?"=w374:bool)
          }
          frame Disabled {
            n165 = Select(t=0.0, s=w403, f=0.2) -> (s? t:f=w400:dbl)
            n166 = Select(t=0.0, s=w388, f=0.2) -> (s? t:f=w389:dbl)
            n167 = Select(t=0.0, s=w391, f=0.2) -> (s? t:f=w390:dbl)
            n168 = Select(t=0.0, s=w392, f=0.2) -> (s? t:f=w393:dbl)
          }
        }
        n169 = global write "Drive_Globals.vi" "Zero_Back_Left"(w369) -> ()
        n170 = global write "Drive_Globals.vi" "Zero_Back_Right"(w364) -> ()
        n171 = global write "Drive_Globals.vi" "Zero_Front_Left"(w362) -> ()
        n172 = global write "Drive_Globals.vi" "Zero_Front_Right"(w357) -> ()
      }
      frame "Write_FR_Position" {
        n173 = global read "Drive_Globals.vi" "FR_Zero"() -> (w404:dbl)
        n174 = global write "Drive_Globals.vi" "FR_Init"(w404) -> ()
        n175 = Build Array(w404) -> (w406:dbl[])
        n176 = call-poly <vilib>:"Write Delimited Spreadsheet.vi"("file path (dialog if empty)"=path "/home/lvuser/natinst/bin/FR_Init.txt" ("file (use dialog)"), "1D data"=w406) -> ()  [unwired: 12 in, 2 out]
      }
      frame "Write_BL_Position" {
        # "s"
        n177 = global read "Drive_Globals.vi" "BL_Zero"() -> (w407:dbl)
        n178 = Build Array(w407) -> (w409:dbl[])
        n179 = global write "Drive_Globals.vi" "BL_Init"(w407) -> ()
        n180 = call-poly <vilib>:"Write Delimited Spreadsheet.vi"("file path (dialog if empty)"=path "/home/lvuser/natinst/bin/BL_Init.txt" ("file (use dialog)"), "1D data"=w409) -> ()  [unwired: 12 in, 2 out]
      }
      frame "Write_BR_Position" {
        n181 = global read "Drive_Globals.vi" "BR_Zero"() -> (w410:dbl)
        n182 = global write "Drive_Globals.vi" "BR_Init"(w410) -> ()
        n183 = Build Array(w410) -> (w412:dbl[])
        n184 = call-poly <vilib>:"Write Delimited Spreadsheet.vi"("file path (dialog if empty)"=path "/home/lvuser/natinst/bin/BR_Init.txt" ("file (use dialog)"), "1D data"=w412) -> ()  [unwired: 12 in, 2 out]
      }
      frame "Distance" {
        w413 = T10 2 items=["PercentOutput"=0, "Position"=1, "Velocity"=2, "Current"=3, "Follower"=5, "MotionProfile"=6, "MotionMagic"=7, "MotionProfileArc"=10, "Disabled"=15] ("Control Mode")
        n185 = call "Command_Drive_Distance.vi"("Startup"=w431, "Distance"=w422, "Timeout"=w423) -> ("Reinit"=w432:bool, "Completed"=w430:bool, "Speeds"=w428:dbl[])  [unwired: 2 in]
        n186 = Send Notification(notification=w430, notifier=w429) -> ()  [unwired: 1 in, 2 out]
        n187 = Index Array(array=w428) -> (element #1=w427:dbl, element #2=w426:dbl, element #3=w425:dbl, element #4=w424:dbl, element #5=w419:dbl, element #6=w421:dbl, element #7=w417:dbl, element #8=w415:dbl)  [unwired: 8 in]
        n188 = call "Drive_Normalize_and_Native_Units.vi"("BR"=w415, "BL"=w417, "FR"=w419, "FL"=w421) -> ("BR_Out"=w414:dbl, "BL_Out"=w416:dbl, "FR_Out"=w418:dbl, "FL_Out"=w420:dbl)
      }
      frame "Time" {
        w440 = T10 2 items=["PercentOutput"=0, "Position"=1, "Velocity"=2, "Current"=3, "Follower"=5, "MotionProfile"=6, "MotionMagic"=7, "MotionProfileArc"=10, "Disabled"=15] ("Control Mode")
        n189 = call "Command_Drive_Time.vi"("Startup"=w436, "Speed_X"=w434, "Speed_Y"=w433, "Timeout"=w435) -> ("Reinit"=w437:bool, "Completed"=w438:bool, "Speeds"=w439:dbl[])  [unwired: 1 in]
        n190 = Send Notification(notification=w438, notifier=w453) -> ()  [unwired: 1 in, 2 out]
        n191 = Index Array(array=w439) -> (element #1=w452:dbl, element #2=w451:dbl, element #3=w450:dbl, element #4=w449:dbl, element #5=w446:dbl, element #6=w448:dbl, element #7=w444:dbl, element #8=w442:dbl)  [unwired: 8 in]
        n192 = call "Drive_Normalize_and_Native_Units.vi"("BR"=w442, "BL"=w444, "FR"=w446, "FL"=w448) -> ("BR_Out"=w441:dbl, "BL_Out"=w443:dbl, "FR_Out"=w445:dbl, "FL_Out"=w447:dbl)
      }
      frame "Turn_To_Heading" {
        w454 = T10 2 items=["PercentOutput"=0, "Position"=1, "Velocity"=2, "Current"=3, "Follower"=5, "MotionProfile"=6, "MotionMagic"=7, "MotionProfileArc"=10, "Disabled"=15] ("Control Mode")
        n193 = call "Command_Turn_To_Heading.vi"("Startup"=w468, "Heading"=w455, "Timeout"=w456) -> ("Reinit"=w469:bool, "Completed"=w467:bool, "Speeds"=w465:dbl[])  [unwired: 2 in]
        n194 = Send Notification(notification=w467, notifier=w466) -> ()  [unwired: 1 in, 2 out]
        n195 = Index Array(array=w465) -> (element #1=w464:dbl, element #2=w463:dbl, element #3=w462:dbl, element #4=w461:dbl, element #5=w460:dbl, element #6=w459:dbl, element #7=w458:dbl, element #8=w457:dbl)  [unwired: 8 in]
      }
      frame "Turn_To_Target" {
        n196 = call "Command_Turn_To_Target.vi"("Startup"=w482, "Timeout"=w470) -> ("Reinit"=w483:bool, "Completed"=w481:bool, "Speeds"=w479:dbl[])  [unwired: 3 in]
        n197 = Send Notification(notification=w481, notifier=w480) -> ()  [unwired: 1 in, 2 out]
        n198 = Index Array(array=w479) -> (element #1=w478:dbl, element #2=w477:dbl, element #3=w476:dbl, element #4=w475:dbl, element #5=w474:dbl, element #6=w473:dbl, element #7=w472:dbl, element #8=w471:dbl)  [unwired: 8 in]
      }
      frame "Drive_To_Target" {
        w486 = T10 2 items=["PercentOutput"=0, "Position"=1, "Velocity"=2, "Current"=3, "Follower"=5, "MotionProfile"=6, "MotionMagic"=7, "MotionProfileArc"=10, "Disabled"=15] ("Control Mode")
        n199 = call "Command_Drive_To_Target.vi"("Startup"=w499, "Speed_Y"=w485, "Allowable_Error"=w484, "Timeout"=w487) -> ("Reinit"=w500:bool, "Completed"=w498:bool, "Speeds"=w496:dbl[])  [unwired: 1 in]
        n200 = Send Notification(notification=w498, notifier=w497) -> ()  [unwired: 1 in, 2 out]
        n201 = Index Array(array=w496) -> (element #1=w495:dbl, element #2=w494:dbl, element #3=w493:dbl, element #4=w492:dbl, element #5=w491:dbl, element #6=w490:dbl, element #7=w489:dbl, element #8=w488:dbl)  [unwired: 8 in]
      }
    }
    n202 = feedback-in #1(w27) -> ()
    n203 = Wait (ms)(milliseconds to wait=u32 35) -> ()  [unwired: 1 out]
    n204 = call <vilib>:"CTRE_Phoenix_MotorControl_Set.vi"("Output"=w67, "Control Mode"=w59, "PhoenixMotorControlDevRef"=w58) -> ()  [unwired: 7 in, 2 out]
    n205 = call <vilib>:"CTRE_Phoenix_MotorControl_Set.vi"("Output"=w65, "Control Mode"=w59, "PhoenixMotorControlDevRef"=w71) -> ()  [unwired: 7 in, 2 out]
    n206 = call <vilib>:"CTRE_Phoenix_MotorControl_Set.vi"("Output"=w61, "Control Mode"=w59, "PhoenixMotorControlDevRef"=w69) -> ()  [unwired: 7 in, 2 out]
    n207 = call <vilib>:"CTRE_Phoenix_MotorControl_Set.vi"("Output"=w63, "Control Mode"=w59, "PhoenixMotorControlDevRef"=w70) -> ()  [unwired: 7 in, 2 out]
    n208 = call <vilib>:"CTRE_Phoenix_MotorControl_Set.vi"("Output"=w60, "Control Mode"=w55, "PhoenixMotorControlDevRef"=w37) -> ()  [unwired: 7 in, 2 out]
    n209 = call <vilib>:"CTRE_Phoenix_MotorControl_Set.vi"("Output"=w62, "Control Mode"=w55, "PhoenixMotorControlDevRef"=w36) -> ()  [unwired: 7 in, 2 out]
    n210 = call <vilib>:"CTRE_Phoenix_MotorControl_Set.vi"("Output"=w66, "Control Mode"=w55, "PhoenixMotorControlDevRef"=w34) -> ()  [unwired: 7 in, 2 out]
    n211 = call <vilib>:"CTRE_Phoenix_MotorControl_Set.vi"("Output"=w64, "Control Mode"=w55, "PhoenixMotorControlDevRef"=w35) -> ()  [unwired: 7 in, 2 out]
  }
